vi "sv_UFF58 Set Abscissa Characteristics.vi"(0 "x-axis units":u16(ring) items=["time"=0, "frequency"=1, "quefrency"=2, "revolutions"=3, "order"=4, "rpm"=11, "rad/s"=21, "index"=65535]) -> (4 "abscissa data characteristics (record 8)":T1={"specific data type"=0, "length units exponent"=0, "force units exponent"=0, "temperature units exponent"=0, "axis label"="NONE", "axis units label"="NONE"} {"specific data type" items=["unknown"=0, "general"=1, "stress"=2, "strain"=3, "temperature"=5, "heat flux"=6, "displacement"=8, "reaction force"=9, "velocity"=11, "acceleration"=12, "excitation force"=13, "pressure"=15, "mass"=16, "time"=17, "frequency"=18, "rpm"=19, "order"=20, "sound pressure"=21, "sound intensity"=22, "sound power"=23]})   [LabVIEW 2017, in "SoundVib_UFF58.lvlib"]
doc: "This VI sets the values of <B>abscissa specific data type</B>, <B>abscissa axis label</B>, and abscissa axis units label</B> in the <B>abscissa data characteristics (record 8)</B>"
uses:
  <vilib>/addons/Sound and Vibration/svt_UFF58/SoundVib_UFF58.lvlib
  <vilib>/addons/Sound and Vibration/svt_UFF58/subVIs/sv_UFF58 Axis Characteristics.ctl
  <vilib>/addons/Sound and Vibration/svt_UFF58/subVIs/sv_UFF58 Specific Datatype.ctl
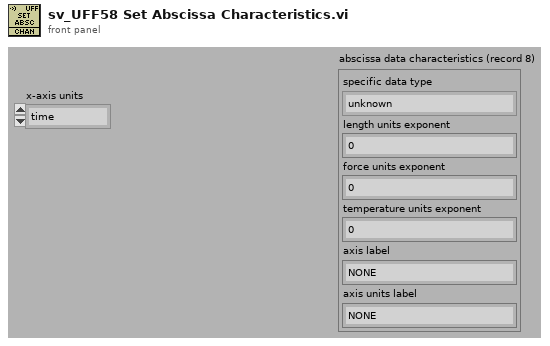
[diagram p1: front panel]
types:
  T1 = typedef "SoundVib_UFF58.lvlib/sv_UFF58 Axis Characteristics.ctl" = cluster{"specific data type":T2, "length units exponent":i32, "force units exponent":i32, "temperature units exponent":i32, "axis label":string, "axis units label":string}
  T2 = typedef "SoundVib_UFF58.lvlib/sv_UFF58 Specific Datatype.ctl" = u16
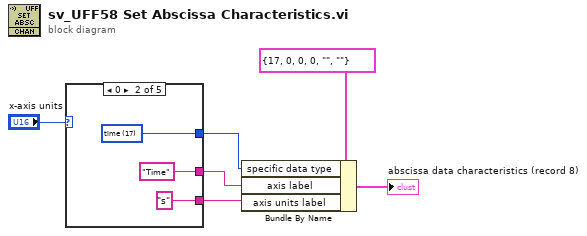
[diagram p0: block diagram]
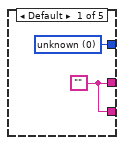
[diagram p2: hidden frame]
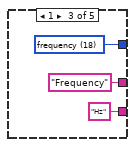
[diagram p3: hidden frame]
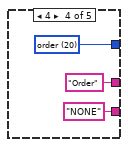
[diagram p4: hidden frame]
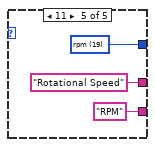
[diagram p5: hidden frame]
diagram:
  n1 = case shown="0" "x-axis units" {
    tunnel: [w8 w11 w14 w17 w20] -> w3
    tunnel: [w7 "Time" ("abscissa axis label") "Frequency" ("abscissa axis label") "Order" ("abscissa axis label") "Rotational Speed" ("abscissa axis label")] -> w2
    tunnel: [w7 "s" ("abscissa axis units label") "Hz" ("abscissa axis units label") "NONE" ("abscissa axis units label") "RPM" ("abscissa axis units label")] -> w1
    frame Default {
      w7 = ""
      w8 = T2 0 items=["unknown"=0, "general"=1, "stress"=2, "strain"=3, "temperature"=5, "heat flux"=6, "displacement"=8, "reaction force"=9, "velocity"=11, "acceleration"=12, "excitation force"=13, "pressure"=15, "mass"=16, "time"=17, "frequency"=18, "rpm"=19, "order"=20, "sound pressure"=21, "sound intensity"=22, "sound power"=23] ("specific data type")
    }
    frame 0 {
      w11 = T2 17 items=["unknown"=0, "general"=1, "stress"=2, "strain"=3, "temperature"=5, "heat flux"=6, "displacement"=8, "reaction force"=9, "velocity"=11, "acceleration"=12, "excitation force"=13, "pressure"=15, "mass"=16, "time"=17, "frequency"=18, "rpm"=19, "order"=20, "sound pressure"=21, "sound intensity"=22, "sound power"=23] ("specific data type")
    }
    frame 1 {
      w14 = T2 18 items=["unknown"=0, "general"=1, "stress"=2, "strain"=3, "temperature"=5, "heat flux"=6, "displacement"=8, "reaction force"=9, "velocity"=11, "acceleration"=12, "excitation force"=13, "pressure"=15, "mass"=16, "time"=17, "frequency"=18, "rpm"=19, "order"=20, "sound pressure"=21, "sound intensity"=22, "sound power"=23] ("specific data type")
    }
    frame 4 {
      w17 = T2 20 items=["unknown"=0, "general"=1, "stress"=2, "strain"=3, "temperature"=5, "heat flux"=6, "displacement"=8, "reaction force"=9, "velocity"=11, "acceleration"=12, "excitation force"=13, "pressure"=15, "mass"=16, "time"=17, "frequency"=18, "rpm"=19, "order"=20, "sound pressure"=21, "sound intensity"=22, "sound power"=23] ("specific data type")
    }
    frame 11 {
      w20 = T2 19 items=["unknown"=0, "general"=1, "stress"=2, "strain"=3, "temperature"=5, "heat flux"=6, "displacement"=8, "reaction force"=9, "velocity"=11, "acceleration"=12, "excitation force"=13, "pressure"=15, "mass"=16, "time"=17, "frequency"=18, "rpm"=19, "order"=20, "sound pressure"=21, "sound intensity"=22, "sound power"=23] ("specific data type")
    }
  }
  n2 = Bundle By Name(cluster=T1 {"specific data type"=17, "length units exponent"=0, "force units exponent"=0, "temperature units exponent"=0, "axis label"="", "axis units label"=""} ("abscissa data characteristics"), "specific data type"=w3, "axis label"=w2, "axis units label"=w1) -> (→"abscissa data characteristics (record 8)":T1)
